vi "Navigation Loop.vi"(8 "error in (no error)":errorcluster) -> (0 "error out":errorcluster)   [LabVIEW 2016]
uses:
  Typedef/INS Data.ctl
  Typedef/UWB Cluster.ctl
  <vilib>/Platform/TimedLoop/XDataNode/wakeup.ctl
  <vilib>/Platform/TimedLoop/XDataNode/XDNodeRunTimeDep.lvlib
  <vilib>/Platform/TimedLoop/XDataNode/nitl_modes.ctl
  <vilib>/Platform/TimedLoop/XDataNode/timing_clust.ctl
  <vilib>/platform/TimedLoop/XDataNode/XDataNode.xnode
  Shared resoruces/gear.vi
  Shared resoruces/Shared resources RT.lvlib
  Shared resoruces/Navigation Variables.vi
  Shared resoruces/ODrive State and Info.vi
  Shared resoruces/Front Panel Control Variables.vi
  <vilib>/ErrorRing/Error Ring.xnode
  <vilib>/Utility/error.llb/Error Cluster From Error Code.vi
  <vilib>/Utility/file.llb/Read Delimited Spreadsheet (DBL).vi
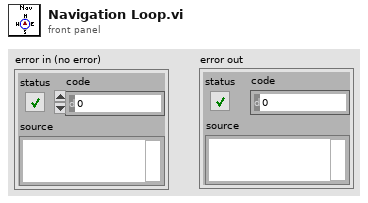
[diagram p1: front panel]
types:
  T1 = typedef "UWB Cluster.ctl" = cluster{"X":dbl, "Y":dbl, "Z":dbl, "heading":dbl, "quality":u8}
  T2 = typedef "INS Data.ctl" = cluster{"Yaw":sgl, "Pitch":sgl, "Roll":sgl, "Lat":dbl, "Long":dbl, "Alt":dbl, "North":dbl, "East":dbl, "Down":dbl, "PosU":dbl, "VelU":dbl}
  T3 = typedef "XDNodeRunTimeDep.lvlib/timing_clust.ctl" = cluster{"Expected End [f-1]":u64, "Actual End [f-1]":u64, "Finished Late? [f-1]":bool, "Expected End [i-1]":u64, "Actual End [i-1]":u64, "Finished Late? [i-1]":bool, "Expected Start [i]":u64, "Actual Start [i]":u64, "Expected Start [f]":u64, "Actual Start [f]":u64, "Source Name":string, "Structure Name":string, "Period":i64, "Deadline":i64, "Offset":i64, "Start":i64, "Priority":i32, "Timeout":i32, "Mode":T4, "Wakeup Reason":T5, "Error":errorcluster, "Source Type":string, "Secondary Source Type":string, "Global End Time":u64, "Global Start Time":u64, "Frame Duration":u64, "Iteration Duration":u64, "Assigned CPU":i32, "I/O Scan Engine Mode":u32}
  T4 = typedef "XDNodeRunTimeDep.lvlib/nitl_modes.ctl" = enum32{"No Change", "Process missed periods, maintain original phase", "Discard missed periods, maintain original phase", "Process missed periods, ignore original phase", "Discard missed periods, ignore original phase"}
  T5 = typedef "XDNodeRunTimeDep.lvlib/wakeup.ctl" = enum32{"Normal", "Aborted", "Asynchronous wakeup", "Timing source error", "Timed loop error", "Timeout"}
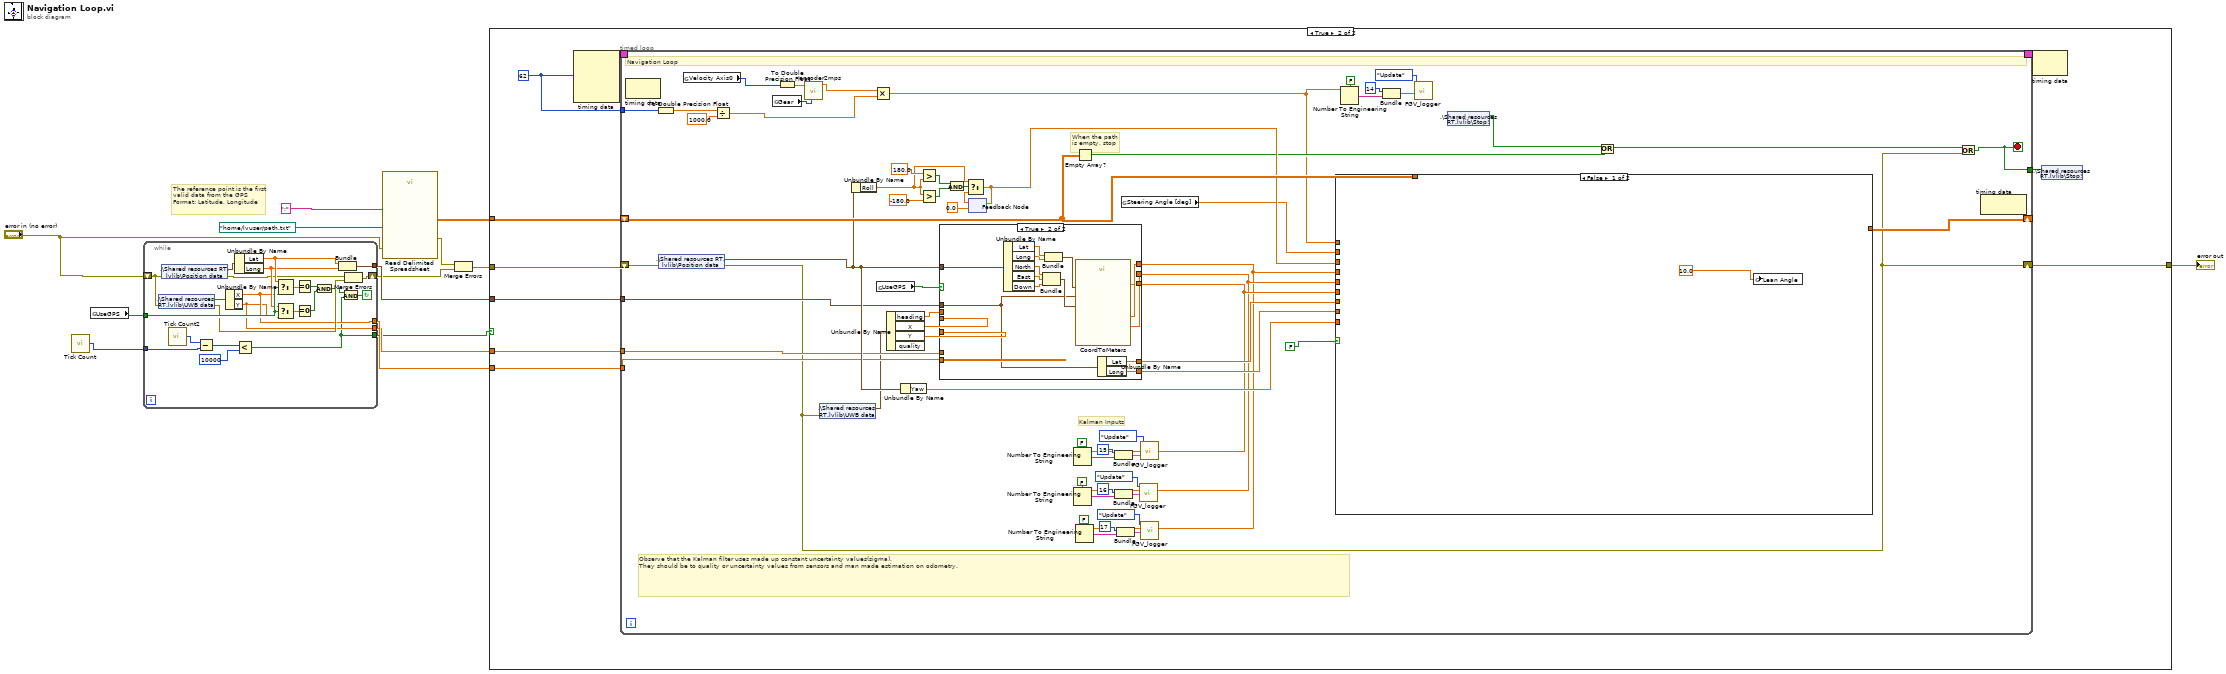
[diagram p0: block diagram]
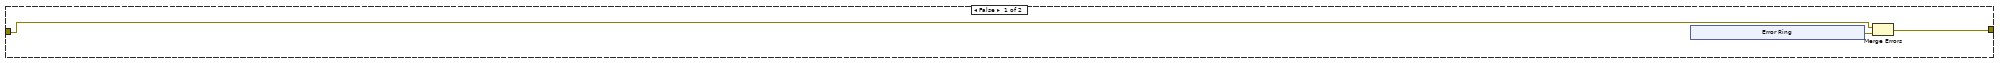
[diagram p2: hidden frame]
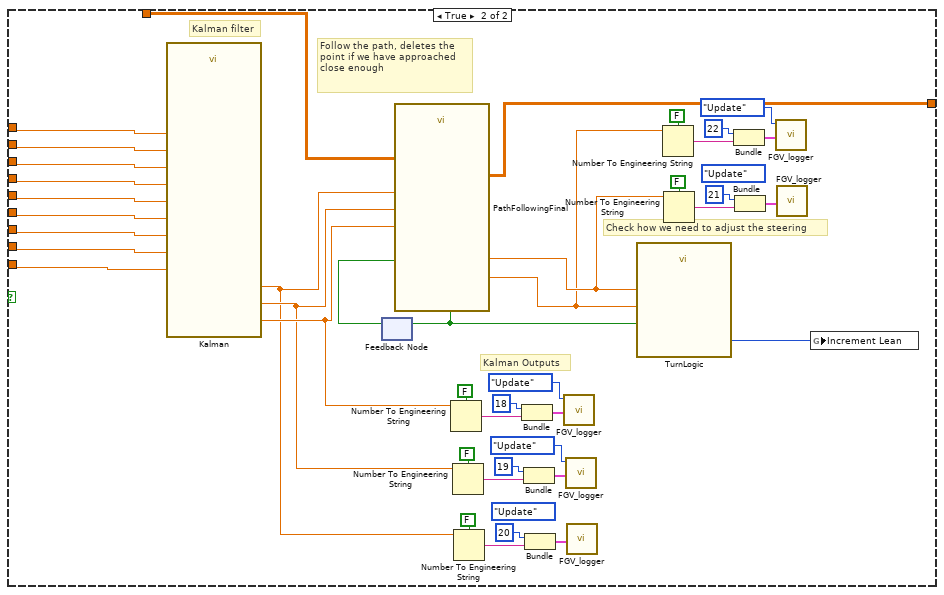
[diagram p3: hidden frame]
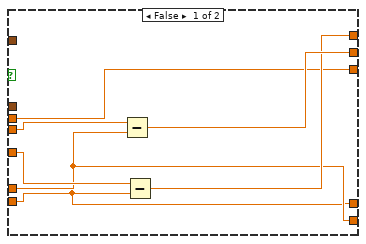
[diagram p4: hidden frame]
diagram:
  # "The reference point is the first valid data from the GPS\nFormat: Latitude, Longitude"
  n1 = call "Tick Count"() -> ("Tick Count(mSec)"=w2:u32)
  n2 = global read "Front Panel Control Variables.vi" "UseGPS"() -> (w12:bool)
  n3 = while {
    shift-right: [w28] -> w6
    shift-left: "error in (no error)" -> [w25]
    tunnel: [w34] -> w9
    tunnel: [w22] -> w10
    tunnel: [w23] -> w11
    tunnel: w12 -> [w32]
    tunnel: w2 -> [w18]
    tunnel: [w15] -> w1
    stop <- w20 continue-if-true
    n4 = shared-variable ".\\Shared resources RT.lvlib\\UWB data"(error in=w25) -> (w24:T1, error out=w26:errorcluster)
    n5 = shared-variable ".\\Shared resources RT.lvlib\\Position data"(error in=w25) -> (w35:T2, error out=w27:errorcluster)
    n6 = call "Tick Count2"() -> ("Tick Count(mSec)"=w19:u32)
    n7 = Subtract(x=w19, y=w18) -> (x-y=w17:u32)
    n8 = Unbundle By Name(w24) -> ("X"=w23:dbl, "Y"=w22:dbl)
    n9 = Unbundle By Name(w35) -> ("Lat"=w31:dbl, "Long"=w30:dbl)
    n10 = Less?(x=w17, y=u32 10000) -> (x < y?=w15:bool)
    n11 = Select(t=w31, s=w32, f=w23) -> (s? t:f=w33:dbl)
    n12 = Select(t=w30, s=w32, f=w22) -> (s? t:f=w29:dbl)
    n13 = Equal To 0?(x=w33) -> (x = 0?=w37:bool)
    n14 = Equal To 0?(x=w29) -> (x = 0?=w36:bool)
    n15 = And(x=w37, y=w36) -> (x .and. y?=w21:bool)
    n16 = Bundle("Lat"=w31, "Long"=w30) -> (w34:cluster{"Lat":dbl, "Long":dbl})  [unwired: 1 in]
    n17 = And(x=w21, y=w15) -> (x .and. y?=w20:bool)
    n18 = Merge Errors(w27, w26) -> (w28:errorcluster)
  }
  n19 = call-poly <vilib>:"Read Delimited Spreadsheet.vi"("file path (dialog if empty)"=path "/home/lvuser/path.txt", "error in (no error)"="error in (no error)", "delimiter (\\t)"=";" ("delimiter (\\t)")) -> ("all rows"=w5:dbl[][], "error out"=w7:errorcluster)  [unwired: 7 in, 4 out]
  n20 = Merge Errors(w7, w6) -> (w8:errorcluster)
  n21 = case shown="True" w1 {
    tunnel: [w38 w53] -> w13
    tunnel: w11 -> [_ w51]
    tunnel: w10 -> [_ w50]
    tunnel: w9 -> [_ w49]
    tunnel: w8 -> [w40 w47]
    tunnel: w5 -> [_ w46]
    frame False {
      n22 = xnode "Error Ring"() -> ("error out"=w39:errorcluster)
      n23 = Merge Errors(w40, w39) -> (w38:errorcluster)
    }
    frame True {
      w52 = i64 62 ("Period")
      n24 = node-c288(w52) -> (w55:T3)  [unwired: 3 in]
      n25 = timed-loop {
        shift-right: [w118] -> _
        shift-left: w46 -> [w117]
        shift-right: [w57] -> w53
        shift-left: w47 -> [w103]
        tunnel: [w99] -> w48
        tunnel: w49 -> [w98]
        tunnel: w50 -> [w97]
        tunnel: w51 -> [w96]
        timing: w55 -> [_]
        timing-out: [_] -> w54
        tunnel: w52 -> [w95]
        stop <- w99 stop-if-true
        # "Observe that the Kalman filter uses made up constant uncertainty values(sigma).\nThey should be to quality or uncertainty values from sensors and man made estimation on odometry."
        # "Kalman Inputs"
        # "When the path is empty, stop"
        # "Navigation Loop"
        n26 = node-c288() -> ()  [unwired: 1 in, 1 out]
        n27 = To Double Precision Float(number=w95) -> (double precision float=w94:dbl)
        n28 = shared-variable ".\\Shared resources RT.lvlib\\Position data"(error in=w103) -> (w104:T2, error out=w57:errorcluster)
        n29 = global read "ODrive State and Info.vi" "Velocity Axis0"() -> (w83:i16)
        n30 = Divide(x=w94, y=1000.0) -> (x/y=w91:dbl)
        n31 = global read "gear.vi" "Gear"() -> (w85:enum16{"7", "6", "5", "4", "3", "2", "1"})
        n32 = To Double Precision Float(number=w83) -> (double precision float=w92:dbl)
        n33 = call "encoder2mps.vi"("Gear"=w85, "encoderSpeed"=w92) -> ("realVelocity"=w90:dbl)  [unwired: 9 in]
        n34 = shared-variable ".\\Shared resources RT.lvlib\\UWB data"(error in=w57) -> (w89:T1)  [unwired: 1 out]
        n35 = Unbundle By Name(w104) -> ("Roll"=w109:sgl)
        n36 = Multiply(x=w90, y=w91) -> (x*y=w66:dbl)
        n37 = global read "Front Panel Control Variables.vi" "UseGPS"() -> (w82:bool)
        n38 = Unbundle By Name(w89) -> ("heading"=w86:dbl, "X"=w88:dbl, "Y"=w87:dbl)  [unwired: 1 out]
        n39 = Unbundle By Name(w104) -> ("Yaw"=w105:sgl)
        n40 = Greater?(x=sgl 180.0 ("upper limit"), y=w109) -> (0:w110:bool)
        n41 = Greater?(x=w109, y=sgl -180.0 ("lower limit")) -> (0:w112:bool)
        n42 = case shown="True" w82 {
          tunnel: [w167 w177] -> w58
          tunnel: [w168 w176] -> w59
          tunnel: [w164 w175] -> w60
          tunnel: [w165 w174] -> w116
          tunnel: [w166 w173] -> w115
          tunnel: w104 -> [_ w172]
          tunnel: w98 -> [_ w171]
          tunnel: w97 -> [w166 _]
          tunnel: w96 -> [w165 _]
          tunnel: w88 -> [w169 _]
          tunnel: w87 -> [w170 _]
          tunnel: w86 -> [w164 _]
          frame False {
            n43 = Subtract(x=w169, y=w166) -> (x-y=w168:dbl)
            n44 = Subtract(x=w170, y=w165) -> (x-y=w167:dbl)
          }
          frame True {
            n45 = Unbundle By Name(w172) -> ("Lat"=w184:dbl, "Long"=w183:dbl, "North"=w181:dbl, "East"=w180:dbl, "Down"=w179:dbl)
            n46 = Bundle("North"=w181, "East"=w180, "Down"=w179) -> (w178:cluster{"North":dbl, "East":dbl, "Down":dbl})  [unwired: 1 in]
            n47 = Bundle("Lat"=w184, "Long"=w183) -> (w182:cluster{"Lat":dbl, "Long":dbl})  [unwired: 1 in]
            n48 = call "CoordToMeters.vi"("VelNed"=w178, "Ref Point"=w171, "GPS position"=w182) -> ("Bike Heading"=w175:dbl, "X"=w176:dbl, "Y"=w177:dbl)  [unwired: 6 in]
            n49 = Unbundle By Name(w171) -> ("Lat"=w174:dbl, "Long"=w173:dbl)
          }
        }
        n50 = And(x=w110, y=w112) -> (x .and. y?=w111:bool)
        n51 = feedback #1(sgl 0.0 ("Roll")) -> (w108:sgl)
        n52 = Select(t=w109, s=w111, f=w108) -> (s? t:f=w106:sgl)
        n53 = feedback-in #1(w106) -> ()
        n54 = Number To Engineering String(1:FALSE ("use system decimal point (T)"), 4:w60) -> (0:w77:string)  [unwired: 2 in]
        n55 = Number To Engineering String(1:FALSE ("use system decimal point (T)"), 4:w59) -> (0:w80:string)  [unwired: 2 in]
        n56 = Number To Engineering String(1:FALSE ("use system decimal point (T)"), 4:w58) -> (0:w61:string)  [unwired: 2 in]
        n57 = Empty Array?(array=w117) -> (empty?=w102:bool)
        n58 = Bundle(15, w77) -> (w76:cluster{i32, string})  [unwired: 1 in]
        n59 = Bundle(16, w80) -> (w79:cluster{i32, string})  [unwired: 1 in]
        n60 = Bundle(17, w61) -> (w62:cluster{i32, string})  [unwired: 1 in]
        n61 = global read "Navigation Variables.vi" "Steering Angle [deg]"() -> (w84:dbl)
        n62 = call "FGV_logger.vi"(9:w79, "Command"=enum16{"Update", "Log", "Init"}."Update") -> ()  [unwired: 9 in, 1 out]
        n63 = call "FGV_logger.vi"(9:w76, "Command"=enum16{"Update", "Log", "Init"}."Update") -> ()  [unwired: 9 in, 1 out]
        n64 = call "FGV_logger.vi"(9:w62, "Command"=enum16{"Update", "Log", "Init"}."Update") -> ()  [unwired: 9 in, 1 out]
        n65 = case shown="False" FALSE {
          tunnel: [_ w161] -> w118
          tunnel: w117 -> [_ w158]
          tunnel: w116 -> [_ w157]
          tunnel: w115 -> [_ w156]
          tunnel: w106 -> [_ w155]
          tunnel: w105 -> [_ w154]
          tunnel: w84 -> [_ w153]
          tunnel: w66 -> [_ w151]
          tunnel: w60 -> [_ w140]
          tunnel: w59 -> [_ w139]
          tunnel: w58 -> [_ w138]
          frame False {
            n66 = global write "Navigation Variables.vi" "Lean Angle"(10.0 ("x")) -> ()
          }
          frame True {
            (unwired) enum16{"Update", "Log", "Init"}."Update" ("Command")
            (unwired) enum16{"Update", "Log", "Init"}."Update" ("Command")
            # "Kalman Outputs"
            # "Check how we need to adjust the steering"
            # "Kalman filter"
            # "Follow the path, deletes the point if we have approached close enough"
            n67 = call "Kalman.vi"("x"=w156, "y"=w157, "theta"=w154, "GPS X"=w139, "GPS Y"=w138, "GPS theta"=w140, "ds"=w151, "phi"=w155, "delta"=w153) -> ("new x"=w132:dbl, "new y"=w131:dbl, "new theta"=w133:dbl)  [unwired: 8 in]
            n68 = feedback #2() -> (w160:bool)  [unwired: 1 in]
            n69 = call "PathFollowingFinal.vi"("GPS_Lat"=w131, "GPS_Long"=w132, "Path"=w158, "Heading angle"=w133, "Save heading"=w160) -> ("Path rest"=w161:dbl[][], "Delta Heading Angle"=w121:dbl, "Goal reached"=w159:bool, "Beta"=w120:dbl)  [unwired: 7 in]
            n70 = feedback-in #2(w159) -> ()
            n71 = Number To Engineering String(1:FALSE ("use system decimal point (T)"), 4:w133) -> (0:w150:string)  [unwired: 2 in]
            n72 = Number To Engineering String(1:FALSE ("use system decimal point (T)"), 4:w132) -> (0:w141:string)  [unwired: 2 in]
            n73 = Number To Engineering String(1:FALSE ("use system decimal point (T)"), 4:w131) -> (0:w134:string)  [unwired: 2 in]
            n74 = Bundle(18, w150) -> (w149:cluster{i32, string})  [unwired: 1 in]
            n75 = Bundle(19, w141) -> (w142:cluster{i32, string})  [unwired: 1 in]
            n76 = Bundle(20, w134) -> (w135:cluster{i32, string})  [unwired: 1 in]
            n77 = call "FGV_logger.vi"(9:w149, "Command"=enum16{"Update", "Log", "Init"}."Update") -> ()  [unwired: 9 in, 1 out]
            n78 = call "FGV_logger.vi"(9:w142, "Command"=enum16{"Update", "Log", "Init"}."Update") -> ()  [unwired: 9 in, 1 out]
            n79 = call "FGV_logger.vi"(9:w135) -> ()  [unwired: 10 in, 1 out]
            n80 = call "TurnLogic.vi"("Goal Reached"=w159, "Beta"=w120, "Delta Theta"=w121) -> ("Increment Lean"=w152:i8)  [unwired: 8 in]
            n81 = Number To Engineering String(1:FALSE ("use system decimal point (T)"), 4:w120) -> (0:w126:string)  [unwired: 2 in]
            n82 = Number To Engineering String(1:FALSE ("use system decimal point (T)"), 4:w121) -> (0:w122:string)  [unwired: 2 in]
            n83 = Bundle(22, w126) -> (w127:cluster{i32, string})  [unwired: 1 in]
            n84 = Bundle(21, w122) -> (w123:cluster{i32, string})  [unwired: 1 in]
            n85 = call "FGV_logger.vi"(9:w127, "Command"=enum16{"Update", "Log", "Init"}."Update") -> ()  [unwired: 9 in, 1 out]
            n86 = call "FGV_logger.vi"(9:w123) -> ()  [unwired: 10 in, 1 out]
            n87 = global write "Navigation Variables.vi" "Increment Lean"(w152) -> ()
          }
        }
        n88 = Number To Engineering String(1:FALSE ("use system decimal point (T)"), 4:w66) -> (0:w74:string)  [unwired: 2 in]
        n89 = Bundle(14, w74) -> (w73:cluster{i32, string})  [unwired: 1 in]
        n90 = call "FGV_logger.vi"(9:w73, "Command"=enum16{"Update", "Log", "Init"}."Update") -> ()  [unwired: 9 in, 1 out]
        n91 = shared-variable ".\\Shared resources RT.lvlib\\Stop!"() -> (w100:bool)  [unwired: 1 in, 1 out]
        n92 = Or(x=w100, y=w102) -> (x .or. y?=w101:bool)
        n93 = Or(x=w101, y=w57) -> (x .or. y?=w99:bool)
        n94 = node-c288() -> ()  [unwired: 1 in, 1 out]
      }
      n95 = node-c288(w54) -> ()  [unwired: 1 out]
      n96 = shared-variable ".\\Shared resources RT.lvlib\\Stop!"(w48) -> ()  [unwired: 1 in, 1 out]
    }
  }
  "error out" <- w13
